vi "QueryFirst_SQL.vi"(4 "TypeMap":refnum<class "TypeMap.lvclass">, 5 "type":refnum<class>, 6 "commandTimeout in":i32=-1, 7 "CommandType":i32(ring)=-1 items=["Text"=1, "StoredProcedure"=4, "TableDirect"=512], 8 "error in (no error)":errorcluster, 9 "Parameters in":variant, 10 "sql":string, 11 "SqlMapper in":refnum<class "SqlMapper.lvclass">) -> (0 "error out":errorcluster, 2 "Value":refnum<class>, 3 "SqlMapper out":refnum<class "SqlMapper.lvclass">)   [LabVIEW 2020, in "ORM_API.lvlib"]
uses:
  ORM_API.lvlib
  <vilib>/Viviota/shared/ORM.lvlibp/ORM/SqlMapper/SqlMapper.lvclass
  <vilib>/Viviota/shared/ORM.lvlibp/ORM/TypeMap/TypeMap.lvclass
  <vilib>/Viviota/shared/ORM.lvlibp/ORM/TypeMap/Create DynamicParameter.vi
  <vilib>/Viviota/shared/ORM.lvlibp/ORM/DynamicParameters/DynamicParameters.lvclass
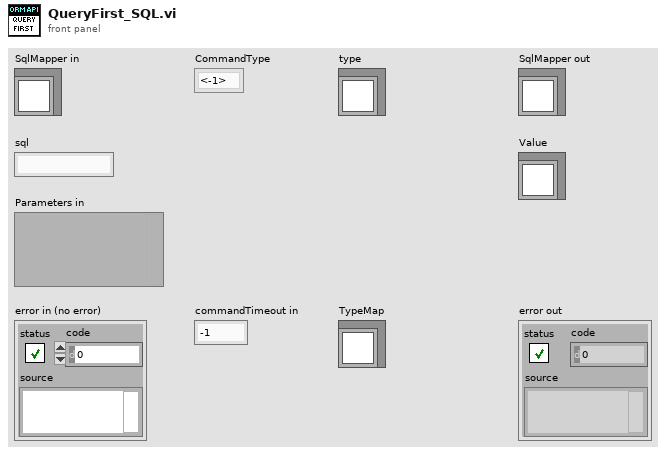
[diagram p1: front panel]
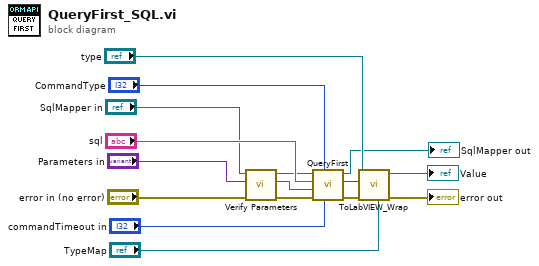
[diagram p0: block diagram]
diagram:
  n1 = call "Verify Parameters.vi"("error in (no error)"="error in (no error)", "Parameters In"="Parameters in", "SqlMapper in"="SqlMapper in") -> ("error out"=w12:errorcluster, "DynamicParameters out"=w10:refnum<class "DynamicParameters.lvclass">, "SqlMapper out"=w8:refnum<class "SqlMapper.lvclass">)  [unwired: 6 in]
  n2 = call-dynamic "QueryFirst.vi"("commandTimeout in"="commandTimeout in", "CommandType"="CommandType", "error in (no error)"=w12, "DynamicParameters in"=w10, "sql"="sql", "SqlMapper in"=w8) -> ("error out"=w7:errorcluster, "Value"=w5:variant, "SqlMapper out"=→"SqlMapper out":refnum<class "SqlMapper.lvclass">)  [unwired: 3 in]
  n3 = call <vilib>:"ToLabVIEW_Wrap.vi"("TypeMap in"="TypeMap", "error in (no error)"=w7, "DbRow"=w5, "TargetObject In"="type") -> ("error out"=→"error out":errorcluster, "Object Out"=→"Value":refnum<class>)  [unwired: 6 in]
